vi "Enstack an Item to Queue1.vi"(8 "Error In":errorcluster, 9 "Add to Queue? (T)":bool=TRUE, 10 "Data":variant, 11 "Item to Add":string) -> (0 "Error Out":errorcluster)   [LabVIEW 2014]
doc: "Adds an item to top of the Queue based on the boolean flag - \"Add to Queue?\"."
uses:
  Typedefs/Queue Type.ctl
  SLL QSM.lvlib
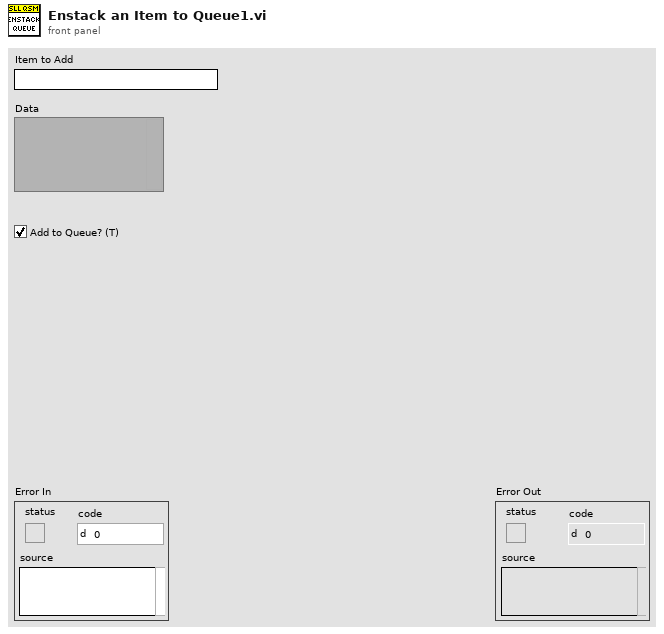
[diagram p1: front panel]
types:
  T1 = typedef "SLL QSM.lvlib/Queue Type.ctl" = cluster{"State":string, "Data":variant}
  T2 = typedef "SLL QSM.lvlib/Queue Reference.ctl" = refnum<queue>
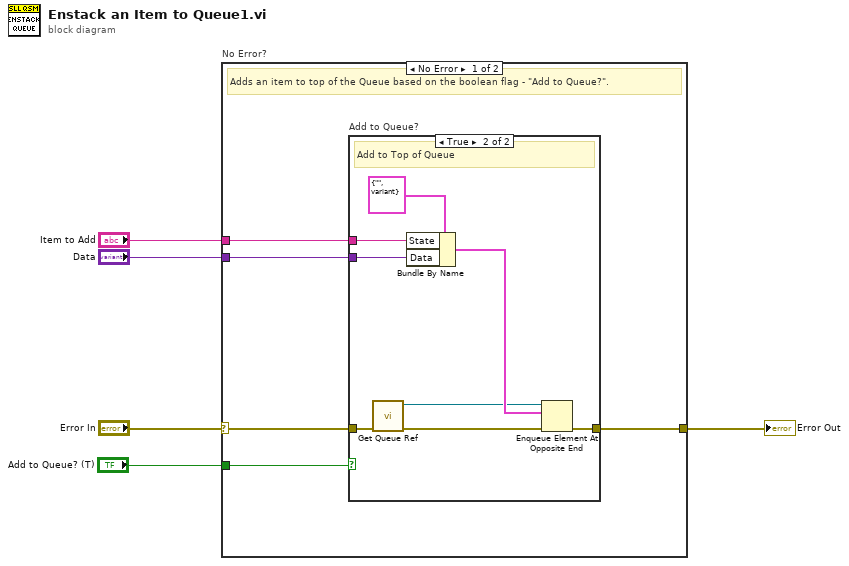
[diagram p0: block diagram]
diagram:
  n1 = case "No Error?" shown="No Error" "Error In" {
    selector: "Error In" -> [w8 w20]
    tunnel: [w10 w20] -> w5
    tunnel: "Item to Add" -> [w9 _]
    tunnel: "Add to Queue? (T)" -> [w7 _]
    tunnel: "Data" -> [w6 _]
    frame No Error {
      # "Adds an item to top of the Queue based on the boolean flag - \"Add to Queue?\"."
      n2 = case "Add to Queue?" shown="True" w7 {
        tunnel: w8 -> [w11 w14]
        tunnel: [w11 w19] -> w10
        tunnel: w9 -> [_ w17]
        tunnel: w6 -> [_ w15]
        frame False {
          # "Skip Adding to Queue"
        }
        frame True {
          # "Add to Top of Queue"
          n3 = call "Get Queue Ref.vi"("Error In"=w14) -> ("Error Out"=w13:errorcluster, "Queue Out"=w12:T2)  [unwired: 9 in]
          n4 = Bundle By Name(cluster=T1 {"State"="", "Data"=variant} ("Queue Type"), "State"=w17, "Data"=w15) -> (w16:T1)
          n5 = Enqueue Element At Opposite End(queue=w12, element=w16, error in (no error)=w13) -> (error out=w19:errorcluster)  [unwired: 1 in, 2 out]
        }
      }
    }
    frame Error {
    }
  }
  "Error Out" <- w5
